vi "Array Type Example.vi"() -> ()   [LabVIEW 2010]
uses:
  Type Defs/File Format.ctl
  Type Defs/Single Tag.ctl
  Type Defs/Data Types.ctl
  Type Defs/Tag Grouping set.ctl
  DataTypes/Array of String_Write.vi
  DataTypes/Array of Boolean_Write.vi
  DataTypes/Array of Double_Write.vi
  DataTypes/Array of Single_Write.vi
  DataTypes/Array of I8_Write.vi
  DataTypes/Array of I16_Write.vi
  DataTypes/Array of I32_Write.vi
  DataTypes/Array of I64_Write.vi
  DataTypes/Array of U8_Write.vi
  DataTypes/Array of U16_Write.vi
  DataTypes/Array of U32_Write.vi
  DataTypes/Array of U64_Write.vi
  DataTypes/Array of Double_Read.vi
  Type to Enum.vi
  DataTypes/Array of String_Type To Enum.vi
  DataTypes/Array of Boolean_Type To Enum.vi
  DataTypes/Array of Double_Type To Enum.vi
  DataTypes/Array of Single_Type To Enum.vi
  DataTypes/Array of I8_Type To Enum.vi
  DataTypes/Array of I16_Type To Enum.vi
  DataTypes/Array of I32_Type To Enum.vi
  DataTypes/Array of I64_Type To Enum.vi
  DataTypes/Array of U8_Type To Enum.vi
  DataTypes/Array of U16_Type To Enum.vi
  DataTypes/Array of U32_Type To Enum.vi
  DataTypes/Array of U64_Type To Enum.vi
  Clear All Memory Blocks.vi
  FGVs/CVT Globals.vi
  FGVs/Tag Memory.vi
  Memory Block.vi
  DataTypes/Array of String_Memory Block.vi
  DataTypes/Array of Boolean_Memory Block.vi
  DataTypes/Array of Double_Memory Block.vi
  DataTypes/Array of Single_Memory Block.vi
  DataTypes/Array of I8_Memory Block.vi
  DataTypes/Array of I16_Memory Block.vi
  DataTypes/Array of I32_Memory Block.vi
  DataTypes/Array of I64_Memory Block.vi
  DataTypes/Array of U8_Memory Block.vi
  DataTypes/Array of U16_Memory Block.vi
  DataTypes/Array of U32_Memory Block.vi
  DataTypes/Array of U64_Memory Block.vi
  DataTypes/Boolean_Memory Block.vi
  DataTypes/String_Memory Block.vi
  DataTypes/U8_Memory Block.vi
  DataTypes/U16_Memory Block.vi
  DataTypes/U32_Memory Block.vi
  DataTypes/U64_Memory Block.vi
  DataTypes/I8_Memory Block.vi
  DataTypes/I16_Memory Block.vi
  DataTypes/I32_Memory Block.vi
  DataTypes/I64_Memory Block.vi
  DataTypes/Single_Memory Block.vi
  DataTypes/Double_Memory Block.vi
  FGVs/Group Memory.vi
  Current Value Table.lvlib
panel:
  out "error out":errorcluster
  out "Value":dbl[](array[numeric])
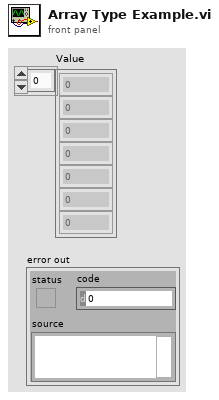
[diagram p1: front panel]
types:
  T1 = typedef "Current Value Table.lvlib/File Format.ctl" = cluster{"Tags":T2[], "Group Listings":T4[]}
  T2 = typedef "Current Value Table.lvlib/Single Tag.ctl" = cluster{"Data Type":T3, "Name":string, "Value":string, "Description":string}
  T3 = typedef "Current Value Table.lvlib/Data Types.ctl" = enum16{"Double", "Single", "I64", "I32", "I16", "I8", "U64", "U32", "U16", "U8", "String", "Boolean", "Array of U8", "Array of U16", "Array of U32", "Array of U64", "Array of I64", "Array of I32", "Array of I16", "Array of I8", "Array of Double", "Array of Single", "Array of Boolean", "Array of String"}
  T4 = typedef "Current Value Table.lvlib/Tag Grouping set.ctl" = cluster{"Group":string, "Tag Names":string[]}
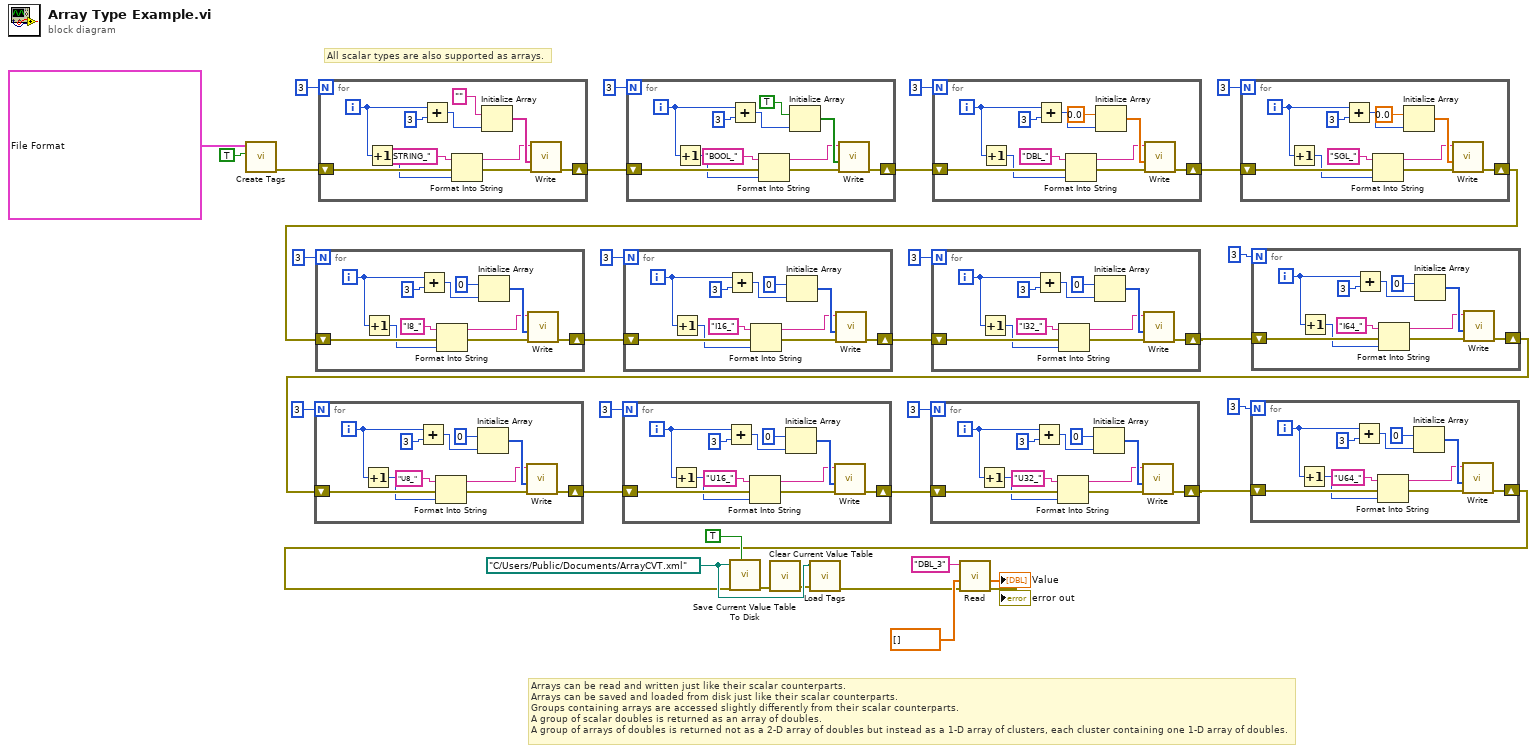
[diagram p0: block diagram]
diagram:
  w4 = path "C:/Users/Public/Documents/ArrayCVT.xml" ("XML File Path")
  # "Arrays can be read and written just like their scalar counterparts.\nArrays can be saved and loaded from disk just like their scalar counterparts.\nGroups containing arrays are accessed slightly differently from their scalar counterparts.\nA group of scalar doubles is returned as an array of doubles.\nA group of arrays of doubles is returned not as a 2-D array of doubles but instead as a 1-D array of clusters, each cluster containing one 1-D array of doubles."
  # "All scalar types are also supported as arrays."
  n1 = call "Create Tags.vi"("Clear Table? (F)"=TRUE ("Clear Engine?"), "CVT Tags to Create"=T1 {"Tags"=[{"Data Type"=enum."Array of U8", "Name"="U8_1", "Value"="", "Description"=""}, {"Data Type"=enum."Array of U8", "Name"="U8_2", "Value"="", "Description"=""}, {"Data Type"=enum."Array of U8", "Name"="U8_3", "Value"="", "Description"=""}, {"Data Type"=enum."Array of U16", "Name"="U16_1", "Value"="", "Description"=""}, {"Data Type"=enum."Array of U16", "Name"="U16_2", "Value"="", "Description"=""}, {"Data Type"=enum."Array of U16", "Name"="U16_3", "Value"="", "Description"=""}, {"Data Type"=enum."Array of U32", "Name"="U32_1", "Value"="", "Description"=""}, {"Data Type"=enum."Array of U32", "Name"="U32_2", "Value"="", "Description"=""}, {"Data Type"=enum."Array of U32", "Name"="U32_3", "Value"="", "Description"=""}, {"Data Type"=enum."Array of U64", "Name"="U64_1", "Value"="", "Description"=""}, {"Data Type"=enum."Array of U64", "Name"="U64_2", "Value"="", "Description"=""}, {"Data Type"=enum."Array of U64", "Name"="U64_3", "Value"="", "Description"=""}, {"Data Type"=enum."Array of I64", "Name"="I64_1", "Value"="", "Description"=""}, {"Data Type"=enum."Array of I64", "Name"="I64_2", "Value"="", "Description"=""}, {"Data Type"=enum."Array of I64", "Name"="I64_3", "Value"="", "Description"=""}, {"Data Type"=enum."Array of I32", "Name"="I32_1", "Value"="", "Description"=""}, {"Data Type"=enum."Array of I32", "Name"="I32_2", "Value"="", "Description"=""}, {"Data Type"=enum."Array of I32", "Name"="I32_3", "Value"="", "Description"=""}, {"Data Type"=enum."Array of I16", "Name"="I16_1", "Value"="", "Description"=""}, {"Data Type"=enum."Array of I16", "Name"="I16_2", "Value"="", "Description"=""}, {"Data Type"=enum."Array of I16", "Name"="I16_3", "Value"="", "Description"=""}, {"Data Type"=enum."Array of I8", "Name"="I8_1", "Value"="", "Description"=""}, {"Data Type"=enum."Array of I8", "Name"="I8_2", "Value"="", "Description"=""}, {"Data Type"=enum."Array of I8", "Name"="I8_3", "Value"="", "Description"=""}, {"Data Type"=enum."Array of Double", "Name"="DBL_1", "Value"="", "Description"=""}, {"Data Type"=enum."Array of Double", "Name"="DBL_2", "Value"="", "Description"=""}, {"Data Type"=enum."Array of Double", "Name"="DBL_3", "Value"="", "Description"=""}, {"Data Type"=enum."Array of Single", "Name"="SGL_1", "Value"="", "Description"=""}, {"Data Type"=enum."Array of Single", "Name"="SGL_2", "Value"="", "Description"=""}, {"Data Type"=enum."Array of Single", "Name"="SGL_3", "Value"="", "Description"=""}, {"Data Type"=enum."Array of Boolean", "Name"="BOOL_1", "Value"="", "Description"=""}, {"Data Type"=enum."Array of Boolean", "Name"="BOOL_2", "Value"="", "Description"=""}, {"Data Type"=enum."Array of Boolean", "Name"="BOOL_3", "Value"="", "Description"=""}, {"Data Type"=enum."Array of String", "Name"="STRING_1", "Value"="", "Description"=""}, {"Data Type"=enum."Array of String", "Name"="STRING_2", "Value"="", "Description"=""}, {"Data Type"=enum."Array of String", "Name"="STRING_3", "Value"="", "Description"=""}], "Group Listings"=[{"Group"="U8", "Tag Names"=["U8_1", "U8_3"]}, {"Group"="U16", "Tag Names"=["U16_1", "U16_2"]}, {"Group"="U32", "Tag Names"=["U32_1", "U32_3"]}, {"Group"="U64", "Tag Names"=["U64_1", "U64_3"]}, {"Group"="I8", "Tag Names"=["I8_1", "I8_3"]}, {"Group"="I16", "Tag Names"=["I16_1", "I16_3"]}, {"Group"="I32", "Tag Names"=["I32_1", "I32_3"]}, {"Group"="I64", "Tag Names"=["I64_1", "I64_3"]}, {"Group"="DBL", "Tag Names"=["DBL_1", "DBL_3"]}, {"Group"="SGL", "Tag Names"=["SGL_1", "SGL_3"]}, {"Group"="BOOL", "Tag Names"=["BOOL_1", "BOOL_3"]}, {"Group"="STRING", "Tag Names"=["STRING_1", "STRING_3"]}]}) -> ("error out"=w21:errorcluster)  [unwired: 9 in]
  n2 = for {
    N: 3 -> [_]
    shift-right: [w44] -> w26
    shift-left: w21 -> [w42]
    i -> [w39]
    n3 = Increment(x=w39) -> (x+1=w38:i32)
    n4 = Add(x=w39, y=3) -> (x+y=w47:i32)
    n5 = Format Into String(initial string="STRING_", error in=w42, w38) -> (resulting string=w40:string, error out=w41:errorcluster)  [unwired: 1 in]
    n6 = Initialize Array("", w47) -> (w45:string[])
    n7 = call-poly "Write.vi"("error in (no error)"=w41, "Value"=w45, "Tag Name"=w40) -> ("error out"=w44:errorcluster)  [unwired: 8 in]
  }
  n8 = for {
    N: 3 -> [_]
    shift-right: [w55] -> w23
    shift-left: w26 -> [w53]
    i -> [w50]
    n9 = Increment(x=w50) -> (x+1=w49:i32)
    n10 = Add(x=w50, y=3) -> (x+y=w58:i32)
    n11 = Format Into String(initial string="BOOL_", error in=w53, w49) -> (resulting string=w51:string, error out=w52:errorcluster)  [unwired: 1 in]
    n12 = Initialize Array(TRUE, w58) -> (w56:bool[])
    n13 = call-poly "Write.vi"("error in (no error)"=w52, "Value"=w56, "Tag Name"=w51) -> ("error out"=w55:errorcluster)  [unwired: 8 in]
  }
  n14 = for {
    N: 3 -> [_]
    shift-right: [w65] -> w32
    shift-left: w23 -> [w63]
    i -> [w60]
    n15 = Increment(x=w60) -> (x+1=w59:i32)
    n16 = Add(x=w60, y=3) -> (x+y=w69:i32)
    n17 = Format Into String(initial string="DBL_", error in=w63, w59) -> (resulting string=w61:string, error out=w62:errorcluster)  [unwired: 1 in]
    n18 = Initialize Array(0.0 ("element"), w69) -> (w67:dbl[])
    n19 = call-poly "Write.vi"("error in (no error)"=w62, "Value"=w67, "Tag Name"=w61) -> ("error out"=w65:errorcluster)  [unwired: 8 in]
  }
  n20 = for {
    N: 3 -> [_]
    shift-right: [w76] -> w22
    shift-left: w32 -> [w74]
    i -> [w71]
    n21 = Increment(x=w71) -> (x+1=w70:i32)
    n22 = Add(x=w71, y=3) -> (x+y=w80:i32)
    n23 = Format Into String(initial string="SGL_", error in=w74, w70) -> (resulting string=w72:string, error out=w73:errorcluster)  [unwired: 1 in]
    n24 = Initialize Array(sgl 0.0 ("element"), w80) -> (w78:sgl[])
    n25 = call-poly "Write.vi"("error in (no error)"=w73, "Value"=w78, "Tag Name"=w72) -> ("error out"=w76:errorcluster)  [unwired: 8 in]
  }
  n26 = for {
    N: 3 -> [_]
    shift-right: [w87] -> w29
    shift-left: w22 -> [w85]
    i -> [w82]
    n27 = Increment(x=w82) -> (x+1=w81:i32)
    n28 = Add(x=w82, y=3) -> (x+y=w91:i32)
    n29 = Format Into String(initial string="I8_", error in=w85, w81) -> (resulting string=w83:string, error out=w84:errorcluster)  [unwired: 1 in]
    n30 = Initialize Array(i8 0 ("element"), w91) -> (w89:i8[])
    n31 = call-poly "Write.vi"("error in (no error)"=w84, "Value"=w89, "Tag Name"=w83) -> ("error out"=w87:errorcluster)  [unwired: 8 in]
  }
  n32 = for {
    N: 3 -> [_]
    shift-right: [w98] -> w27
    shift-left: w29 -> [w96]
    i -> [w93]
    n33 = Increment(x=w93) -> (x+1=w92:i32)
    n34 = Add(x=w93, y=3) -> (x+y=w102:i32)
    n35 = Format Into String(initial string="I16_", error in=w96, w92) -> (resulting string=w94:string, error out=w95:errorcluster)  [unwired: 1 in]
    n36 = Initialize Array(i16 0 ("element"), w102) -> (w100:i16[])
    n37 = call-poly "Write.vi"("error in (no error)"=w95, "Value"=w100, "Tag Name"=w94) -> ("error out"=w98:errorcluster)  [unwired: 8 in]
  }
  n38 = for {
    N: 3 -> [_]
    shift-right: [w109] -> w19
    shift-left: w27 -> [w107]
    i -> [w104]
    n39 = Increment(x=w104) -> (x+1=w103:i32)
    n40 = Add(x=w104, y=3) -> (x+y=w113:i32)
    n41 = Format Into String(initial string="I32_", error in=w107, w103) -> (resulting string=w105:string, error out=w106:errorcluster)  [unwired: 1 in]
    n42 = Initialize Array(0 ("element"), w113) -> (w111:i32[])
    n43 = call-poly "Write.vi"("error in (no error)"=w106, "Value"=w111, "Tag Name"=w105) -> ("error out"=w109:errorcluster)  [unwired: 8 in]
  }
  n44 = for {
    N: 3 -> [_]
    shift-right: [w120] -> w11
    shift-left: w19 -> [w118]
    i -> [w115]
    n45 = Increment(x=w115) -> (x+1=w114:i32)
    n46 = Add(x=w115, y=3) -> (x+y=w124:i32)
    n47 = Format Into String(initial string="I64_", error in=w118, w114) -> (resulting string=w116:string, error out=w117:errorcluster)  [unwired: 1 in]
    n48 = Initialize Array(i64 0 ("element"), w124) -> (w122:i64[])
    n49 = call-poly "Write.vi"("error in (no error)"=w117, "Value"=w122, "Tag Name"=w116) -> ("error out"=w120:errorcluster)  [unwired: 8 in]
  }
  n50 = for {
    N: 3 -> [_]
    shift-right: [w131] -> w14
    shift-left: w11 -> [w129]
    i -> [w126]
    n51 = Increment(x=w126) -> (x+1=w125:i32)
    n52 = Add(x=w126, y=3) -> (x+y=w135:i32)
    n53 = Format Into String(initial string="U8_", error in=w129, w125) -> (resulting string=w127:string, error out=w128:errorcluster)  [unwired: 1 in]
    n54 = Initialize Array(u8 0 ("element"), w135) -> (w133:u8[])
    n55 = call-poly "Write.vi"("error in (no error)"=w128, "Value"=w133, "Tag Name"=w127) -> ("error out"=w131:errorcluster)  [unwired: 8 in]
  }
  n56 = for {
    N: 3 -> [_]
    shift-right: [w142] -> w16
    shift-left: w14 -> [w140]
    i -> [w137]
    n57 = Increment(x=w137) -> (x+1=w136:i32)
    n58 = Add(x=w137, y=3) -> (x+y=w146:i32)
    n59 = Format Into String(initial string="U16_", error in=w140, w136) -> (resulting string=w138:string, error out=w139:errorcluster)  [unwired: 1 in]
    n60 = Initialize Array(u16 0 ("element"), w146) -> (w144:u16[])
    n61 = call-poly "Write.vi"("error in (no error)"=w139, "Value"=w144, "Tag Name"=w138) -> ("error out"=w142:errorcluster)  [unwired: 8 in]
  }
  n62 = for {
    N: 3 -> [_]
    shift-right: [w153] -> w18
    shift-left: w16 -> [w151]
    i -> [w148]
    n63 = Increment(x=w148) -> (x+1=w147:i32)
    n64 = Add(x=w148, y=3) -> (x+y=w157:i32)
    n65 = Format Into String(initial string="U32_", error in=w151, w147) -> (resulting string=w149:string, error out=w150:errorcluster)  [unwired: 1 in]
    n66 = Initialize Array(u32 0 ("element"), w157) -> (w155:u32[])
    n67 = call-poly "Write.vi"("error in (no error)"=w150, "Value"=w155, "Tag Name"=w149) -> ("error out"=w153:errorcluster)  [unwired: 8 in]
  }
  n68 = for {
    N: 3 -> [_]
    shift-right: [w164] -> w1
    shift-left: w18 -> [w162]
    i -> [w159]
    n69 = Increment(x=w159) -> (x+1=w158:i32)
    n70 = Add(x=w159, y=3) -> (x+y=w168:i32)
    n71 = Format Into String(initial string="U64_", error in=w162, w158) -> (resulting string=w160:string, error out=w161:errorcluster)  [unwired: 1 in]
    n72 = Initialize Array(u64 0 ("element"), w168) -> (w166:u64[])
    n73 = call-poly "Write.vi"("error in (no error)"=w161, "Value"=w166, "Tag Name"=w160) -> ("error out"=w164:errorcluster)  [unwired: 8 in]
  }
  n74 = call "Save Current Value Table To Disk.vi"("Force Lookup? (F)"=TRUE, "error in (no error)"=w1, "XML File Path"=w4) -> ("error out"=w3:errorcluster)  [unwired: 8 in]
  n75 = call "Clear Current Value Table.vi"("error in (no error)"=w3) -> ("error out"=w2:errorcluster)  [unwired: 10 in]
  n76 = call "Load Tags.vi"("error in (no error)"=w2, "XML File Path"=w4) -> ("error out"=w5:errorcluster)  [unwired: 8 in, 1 out]
  n77 = call-poly "Read.vi"("error in (no error)"=w5, "Default"=dbl[] [], "Tag Name"="DBL_3") -> ("error out"=→"error out":errorcluster, "Value"=→"Value":dbl[])  [unwired: 7 in]
